vi "Keyence handler.vi"(8 "error in (no error)":errorcluster, 11 "Message Queues out":T3) -> (0 "error out":errorcluster, 3 "Message Queue":refnum<queue>)   [LabVIEW 2014]
uses:
  support/Message Queue/All Message Queues.ctl
  support/Message Queue/Message Cluster.ctl
  Keyence data cluster.ctl
  Keyence Status.ctl
  support/Message Queue/Lossy Enqueue Message (Single).vi
  support/Message Queue/Enqueue Message (Single).vi
  <vilib>/Utility/error.llb/Error Cluster From Error Code.vi
  <vilib>/ErrorRing/Error Ring.xnode
  support/Message Queue/Message Queue.lvlib
panel:
  in  "MBActX":refnum<k7>(container)
  out "Keyence Data Cluster":T1
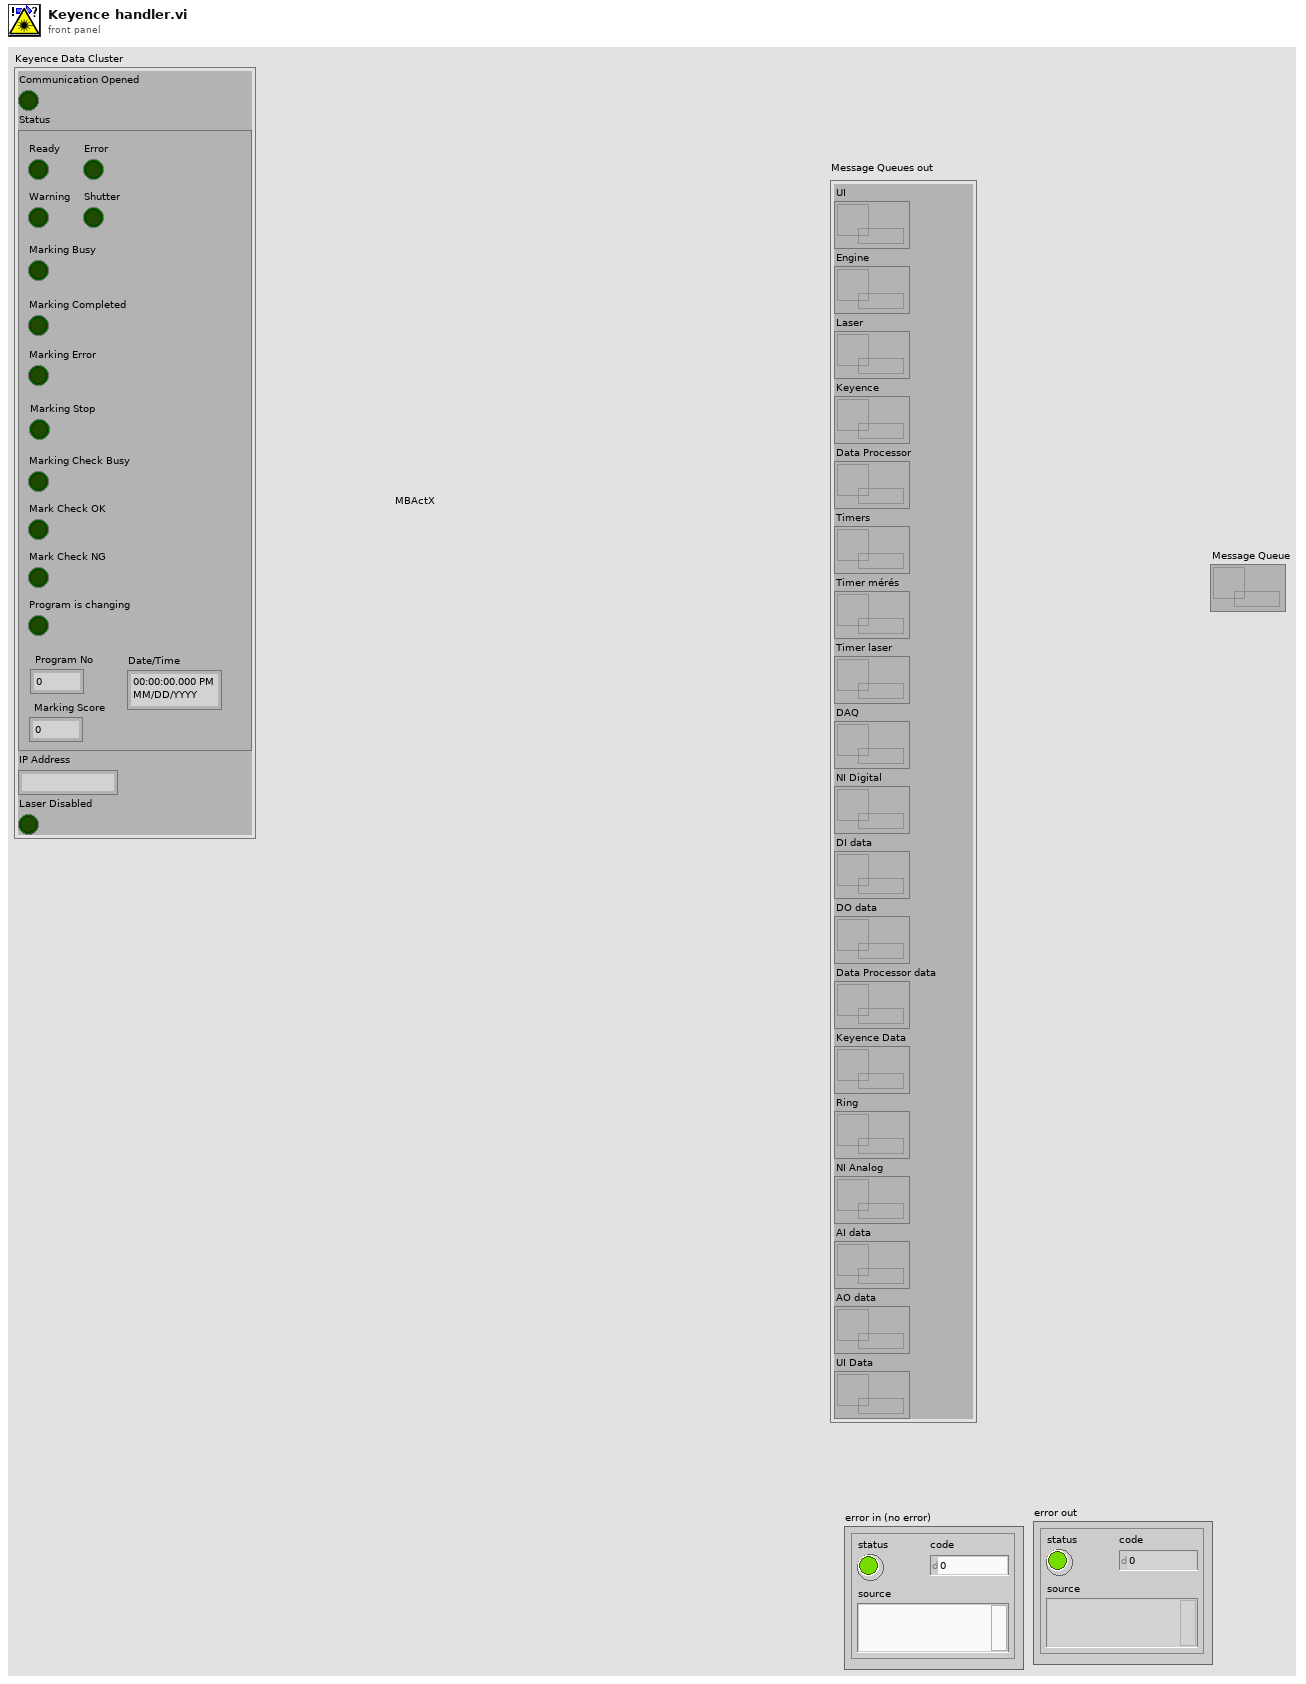
[diagram p1: front panel]
types:
  T1 = typedef "Keyence data cluster.ctl" = cluster{"Communication Opened":bool, "Status":T2, "IP Address":string, "Laser Disabled":bool}
  T2 = typedef "Keyence Status.ctl" = cluster{"Ready":bool, "Error":bool, "Warning":bool, "Shutter":bool, "Mark Check OK":bool, "Mark Check NG":bool, "Marking Busy":bool, "Program No":u16, "Marking Check Busy":bool, "Marking Completed":bool, "Marking Score":u16, "Marking Error":bool, "Marking Stop":bool, "Program is changing":bool, "Date/Time":timestamp}
  T3 = typedef "Message Queue.lvlib/All Message Queues.ctl" = cluster{"UI":refnum<queue>, "Engine":refnum<queue>, "Laser":refnum<queue>, "Keyence":refnum<queue>, "Data Processor":refnum<queue>, "Timers":refnum<queue>, "Timer mérés":refnum<queue>, "Timer laser":refnum<queue>, "DAQ":refnum<queue>, "NI Digital":refnum<queue>, "DI data":refnum<queue>, "DO data":refnum<queue>, "Data Processor data":refnum<queue>, "Keyence Data":refnum<queue>, "Ring":refnum<queue>, "NI Analog":refnum<queue>, "AI data":refnum<queue>, "AO data":refnum<queue>, "UI Data":refnum<queue>}
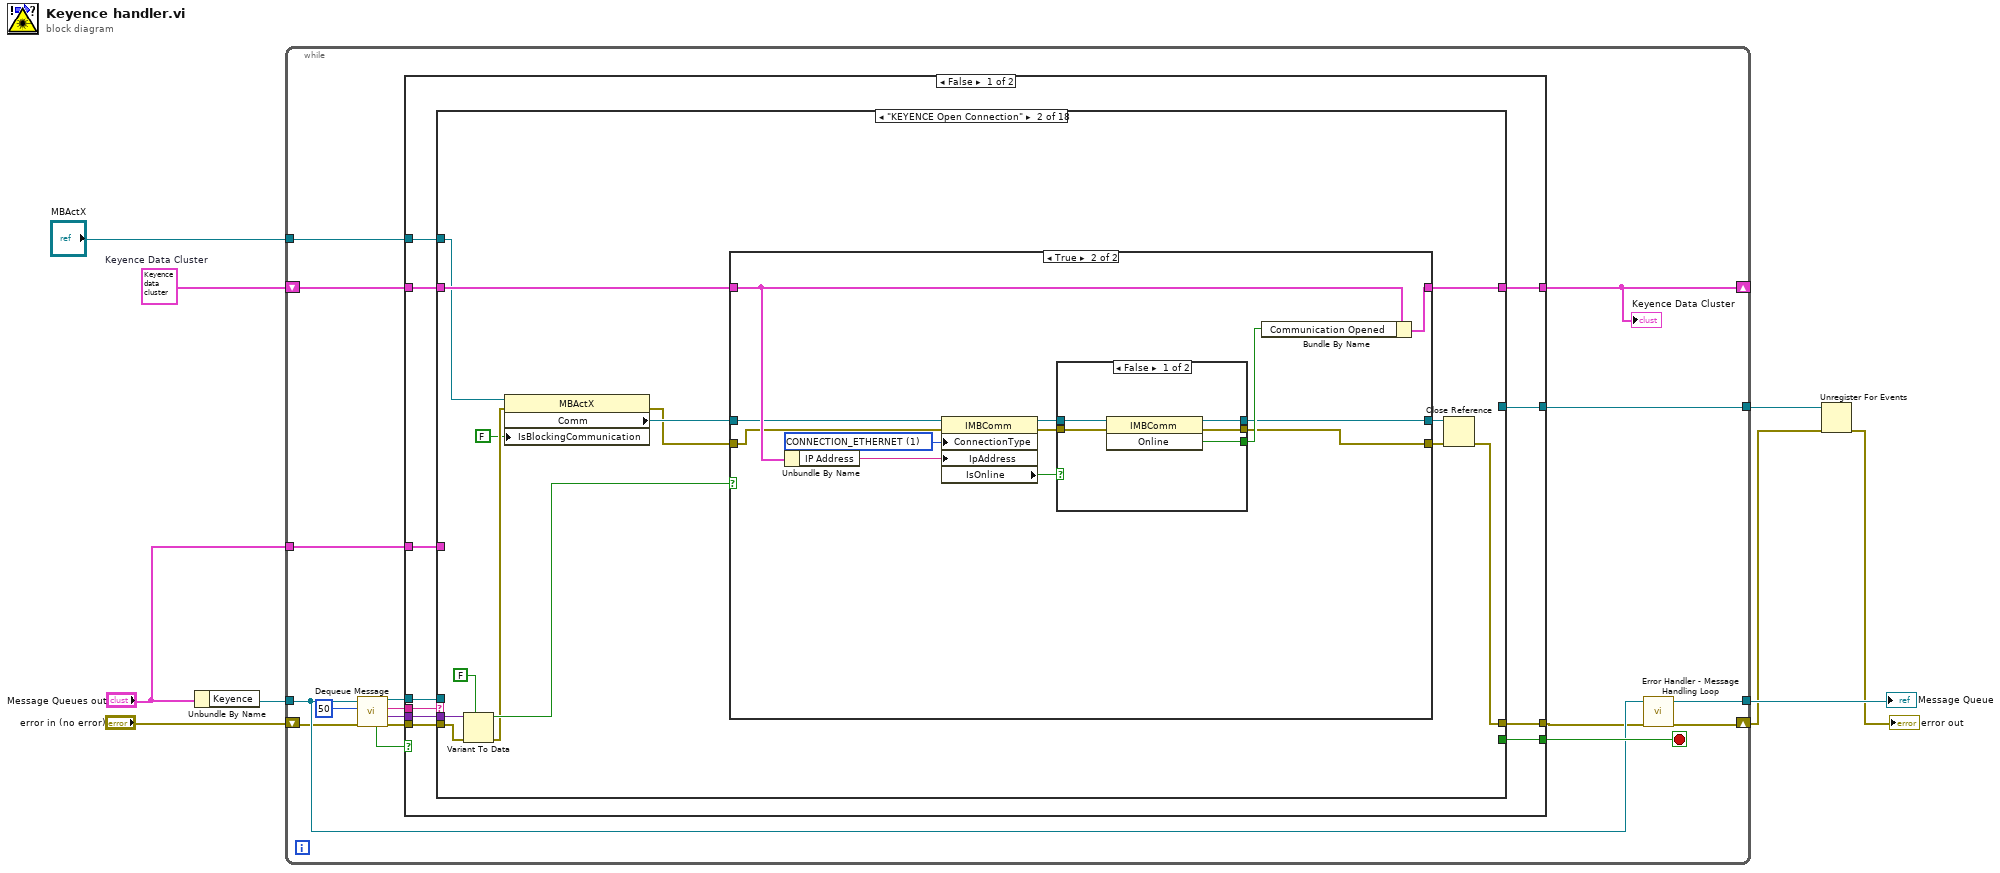
[diagram p0: block diagram]
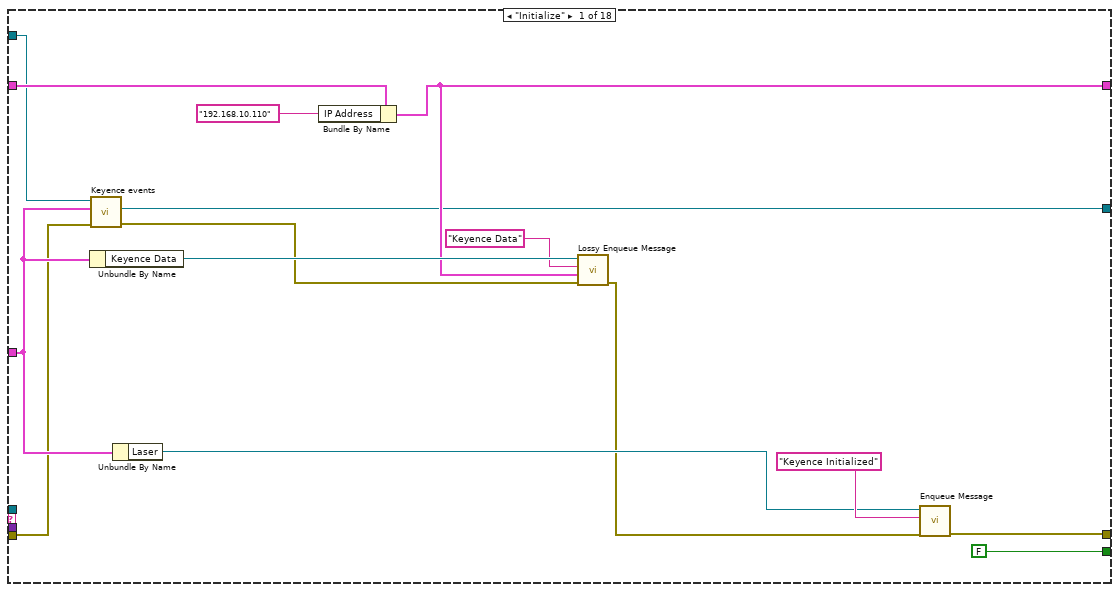
[diagram p2: hidden frame]
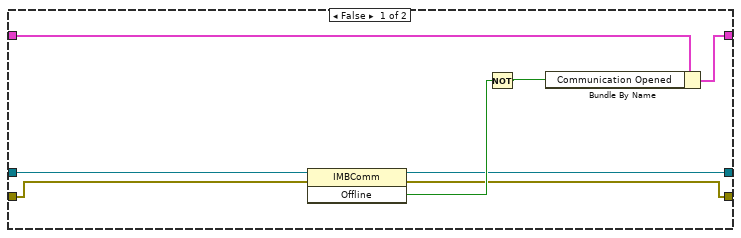
[diagram p3: hidden frame]
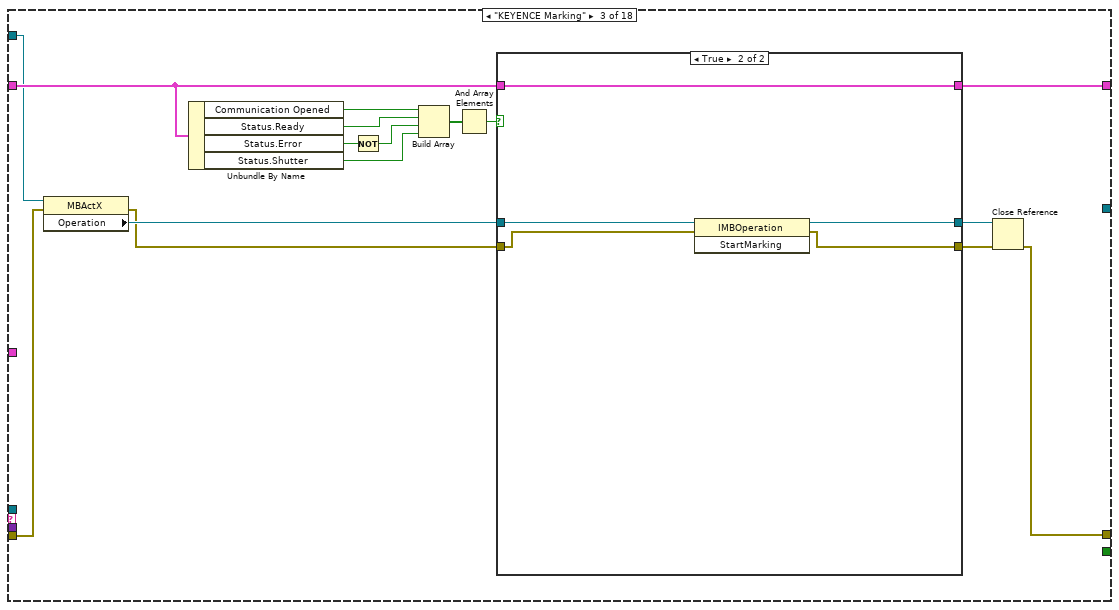
[diagram p5: hidden frame]
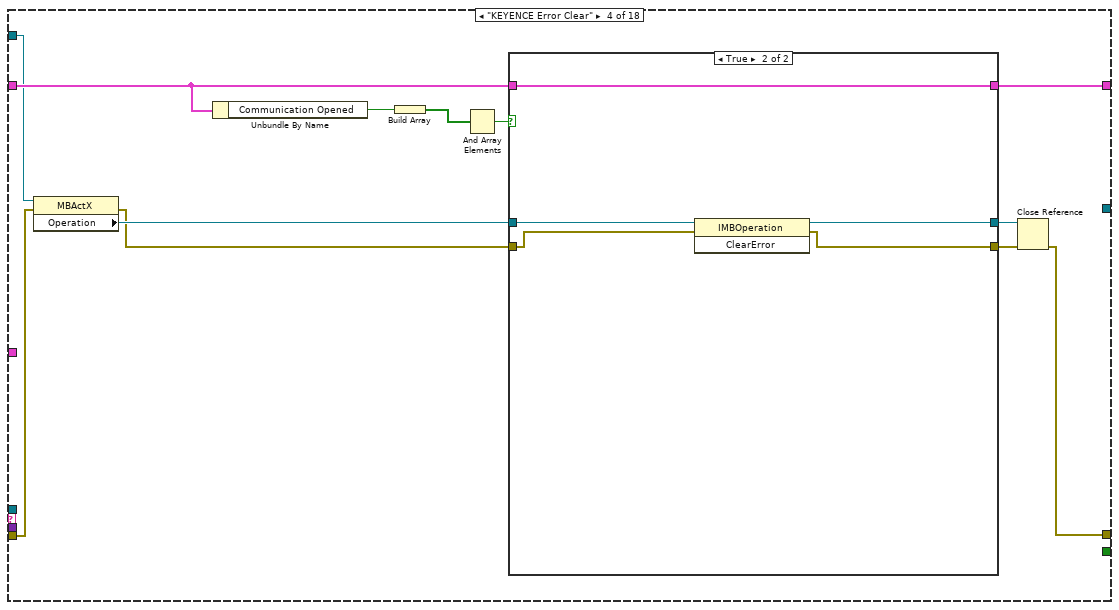
[diagram p7: hidden frame]
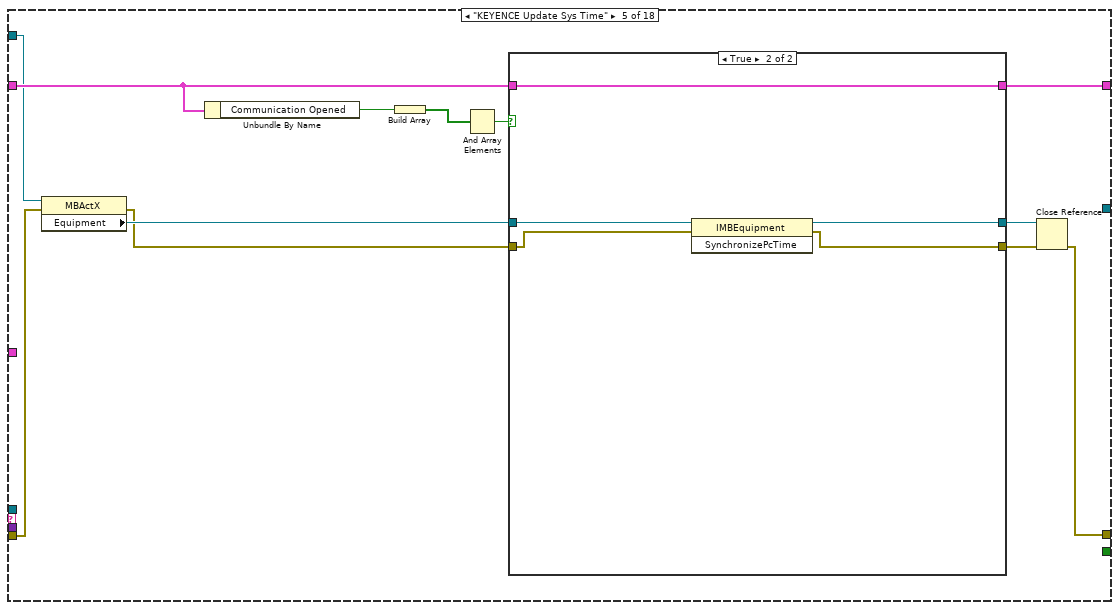
[diagram p9: hidden frame]
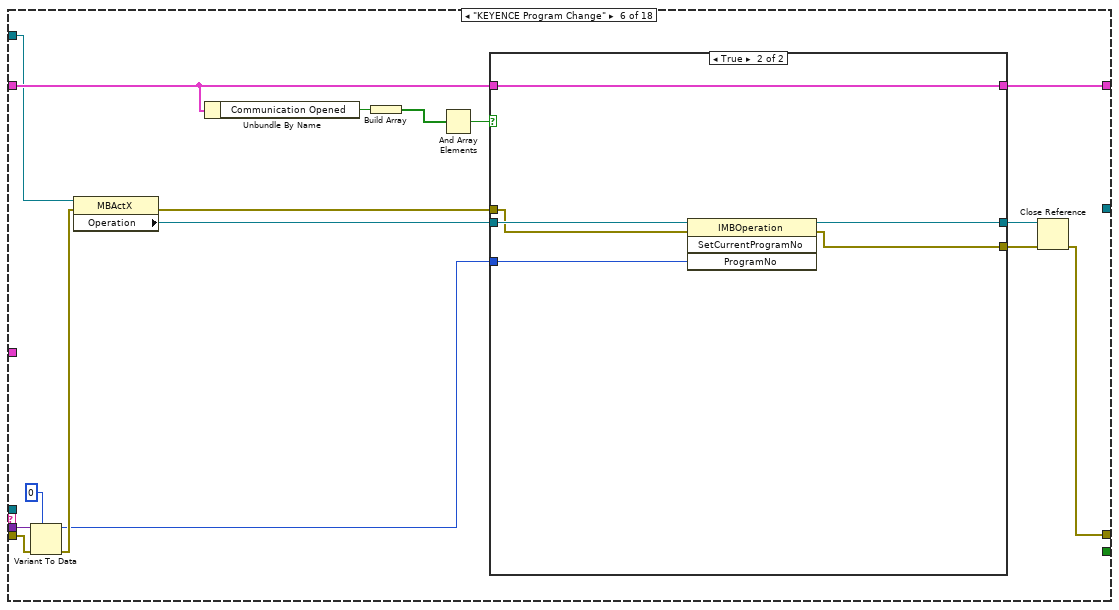
[diagram p11: hidden frame]
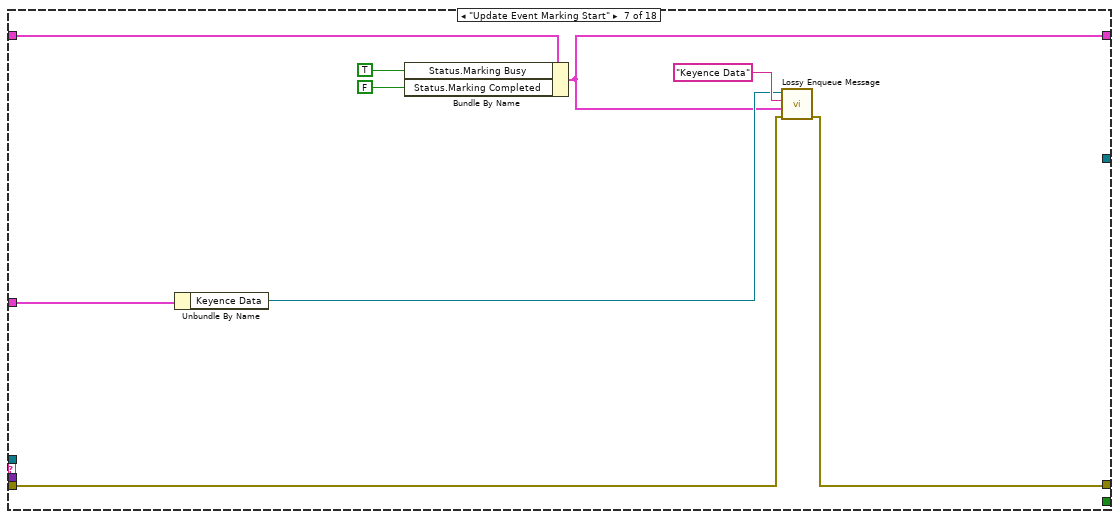
[diagram p13: hidden frame]
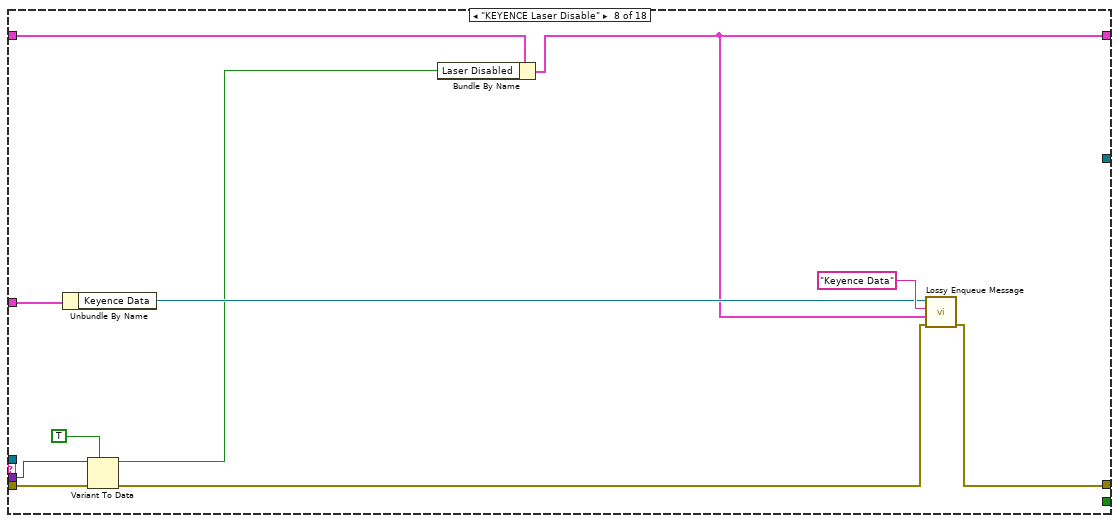
[diagram p14: hidden frame]
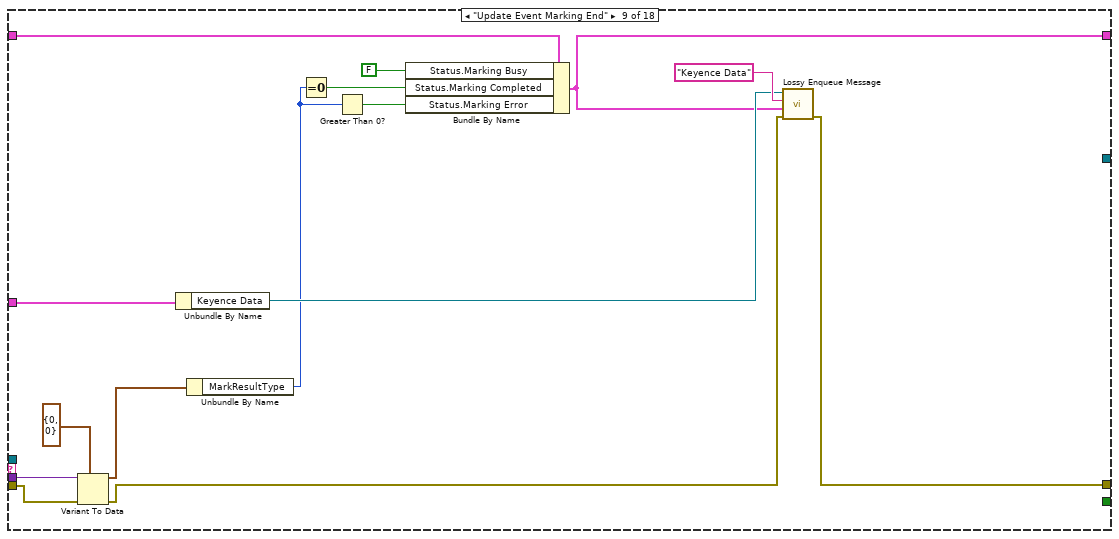
[diagram p15: hidden frame]
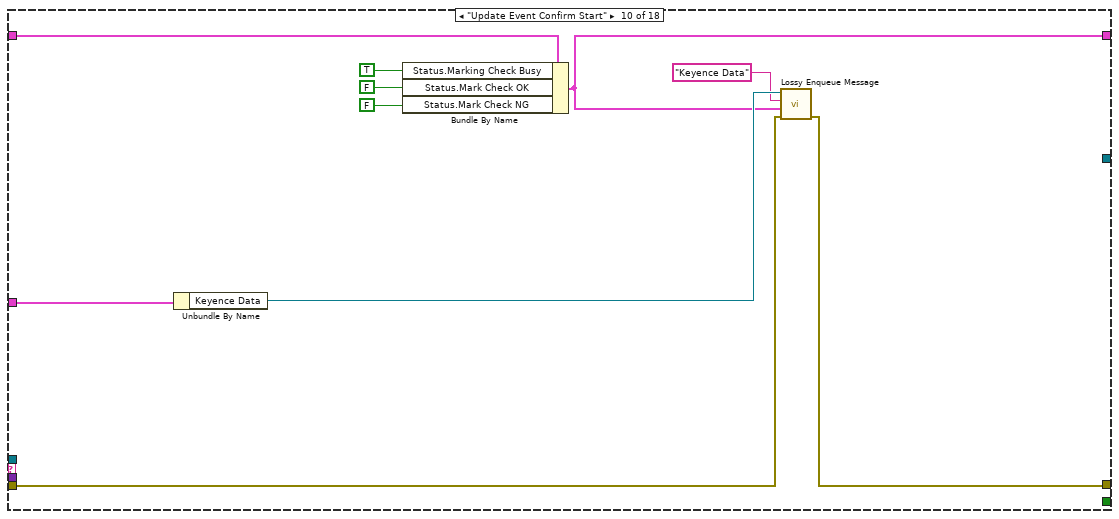
[diagram p16: hidden frame]
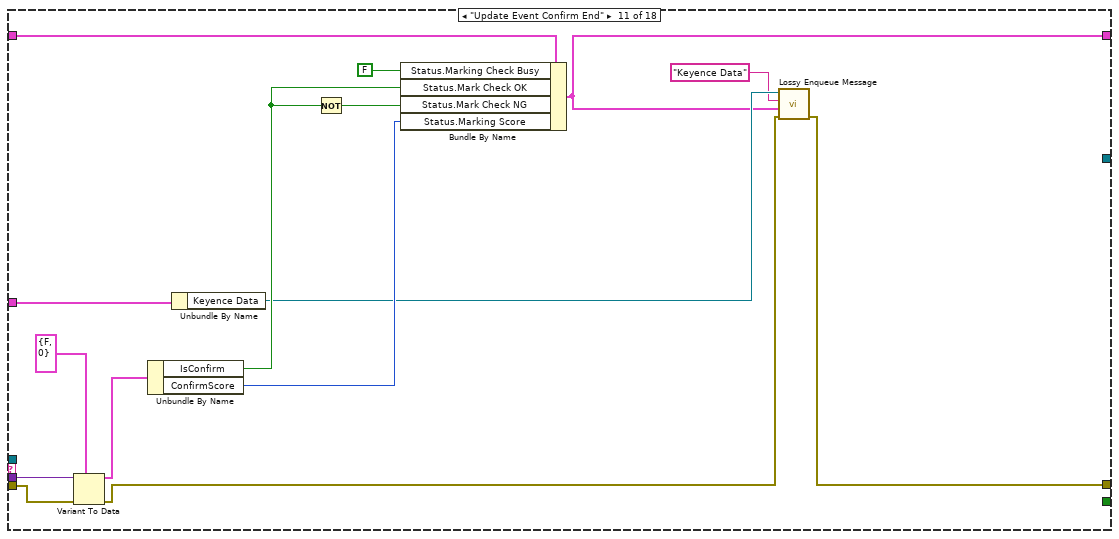
[diagram p17: hidden frame]
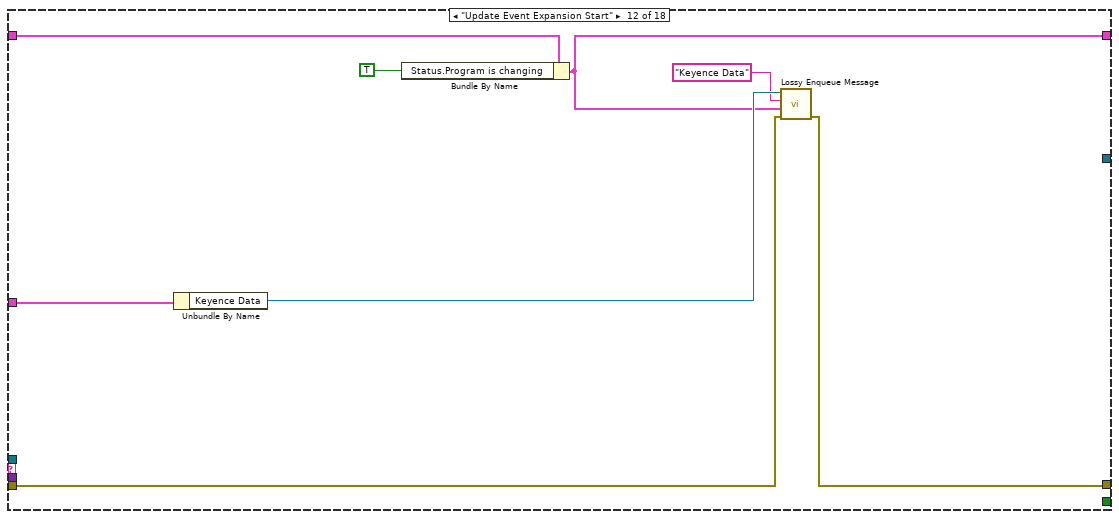
[diagram p18: hidden frame]
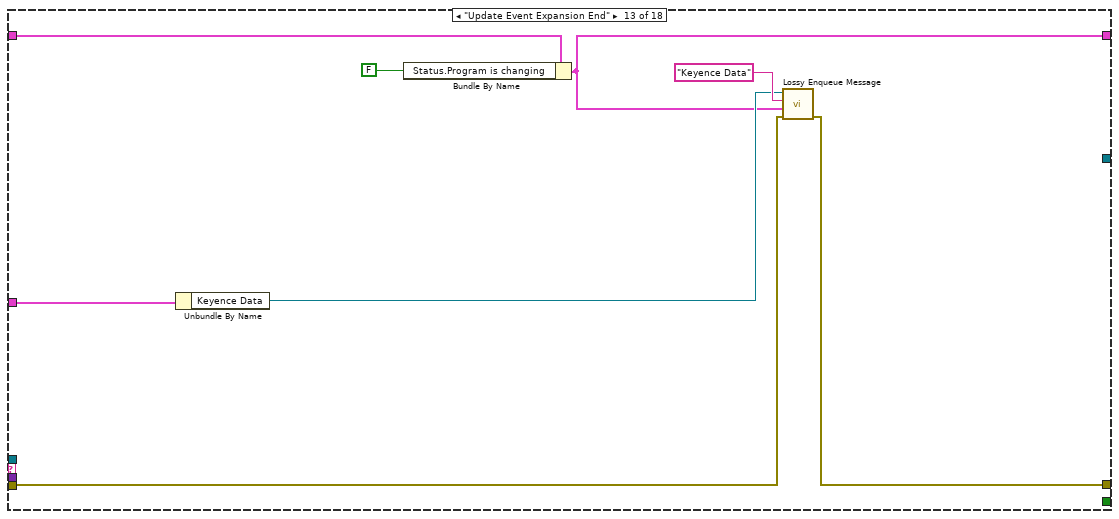
[diagram p19: hidden frame]
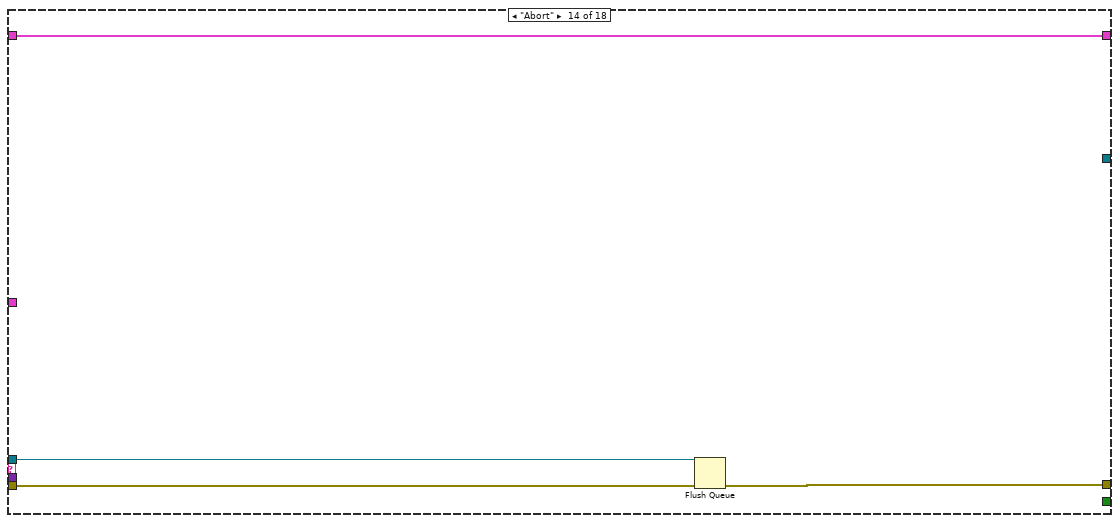
[diagram p20: hidden frame]
diagram:
  w6 = T1 {"Communication Opened"=FALSE, "Status"={"Ready"=FALSE, "Error"=FALSE, "Warning"=FALSE, "Shutter"=FALSE, "Mark Check OK"=FALSE, "Mark Check NG"=FALSE, "Marking Busy"=FALSE, "Program No"=0, "Marking Check Busy"=FALSE, "Marking Completed"=FALSE, "Marking Score"=0, "Marking Error"=FALSE, "Marking Stop"=FALSE, "Program is changing"=FALSE, "Date/Time"=timestamp(0 s since 1904-01-01)}, "IP Address"="", "Laser Disabled"=FALSE}  # Keyence Data Cluster
  n1 = Unbundle By Name("Message Queues out") -> ("Keyence"=w8:refnum<queue>)
  n2 = while {
    tunnel: w8 -> [w16]
    shift-right: [w15] -> _
    shift-left: w6 -> [w14]
    shift-right: [w19] -> w1
    shift-left: "error in (no error)" -> [w12]
    tunnel: "Message Queues out" -> [w18]
    tunnel: [w17] -> w7
    tunnel: [w13] -> w4
    tunnel: "MBActX" -> [w10]
    stop <- w23 stop-if-true
    n3 = call "Dequeue Message.vi"("error in (no error)"=w12, "timeout in ms (-1)"=50, "Message Queue"=w16) -> ("error out"=w25:errorcluster, "Message Data"=w20:variant, "Message"=w26:string, "dup Message Queue"=w24:refnum<queue>, "timed out?"=w21:bool)  [unwired: 4 in]
    n4 = case shown="False" w21 {
      tunnel: w26 -> [w37 _]
      tunnel: w25 -> [w36 w311]
      tunnel: w24 -> [w35 _]
      tunnel: [w34 FALSE] -> w23
      tunnel: [w33 w312] -> w11
      tunnel: w14 -> [w32 w310]
      tunnel: [w29 w306] -> w15
      tunnel: w20 -> [w31 _]
      tunnel: w18 -> [w30 w308]
      tunnel: w10 -> [w28 w304]
      tunnel: [w27 _] -> w13
      frame False {
        n5 = case shown="\"KEYENCE Open Connection\"" w37 {
          selector: w37 -> [_ _ _ _ _ _ _ _ _ _ _ _ _ _ _ _ _ w293]
          tunnel: w36 -> [w41 w63 w101 w125 w145 w167 w185 w196 w206 w220 w231 w245 w253 w263 w265 w279 w282 _]
          tunnel: w35 -> [_ _ _ _ _ _ _ _ _ _ _ _ _ w262 w268 w278 w292 _]
          tunnel: [w51 w54 w98 w121 w141 w161 w184 w198 w204 w219 w229 w244 w252 w260 w269 w280 w283 w294] -> w33
          tunnel: [FALSE _ _ _ _ _ _ _ _ _ _ _ _ _ _ _ TRUE FALSE] -> w34
          tunnel: w32 -> [w48 w62 w109 w129 w149 w173 w188 w201 w210 w223 w235 w248 w256 w261 w264 w281 w290 w296]
          tunnel: w31 -> [_ w64 _ _ _ w168 _ w195 w207 _ w232 _ _ _ w266 _ _ _]
          tunnel: w30 -> [w42 _ _ _ _ _ w186 w199 w208 w221 w233 w246 w254 _ w267 _ w285 _]
          tunnel: [w44 w61 w110 w130 w150 w174 w187 w200 w209 w222 w234 w247 w255 w261 w264 w281 w290 w296] -> w29
          tunnel: w28 -> [w38 w57 w100 w124 w144 w164 _ _ _ _ _ _ _ _ _ _ _ _]
          tunnel: [w39 _ _ _ _ _ _ _ _ _ _ _ _ _ _ _ _ _] -> w27
          frame "Initialize" {
            n6 = Unbundle By Name(w42) -> ("Keyence Data"=w46:refnum<queue>)
            n7 = call "Keyence events.vi"("error in"=w41, "Variant"=w42, "Automation Refnum in"=w38) -> ("error out"=w40:errorcluster, "event callback refnum"=w39:refnum<k27>)  [unwired: 7 in]
            n8 = Unbundle By Name(w42) -> ("Laser"=w49:refnum<queue>)
            n9 = Bundle By Name(cluster=w48, "IP Address"="192.168.10.110" ("Ethernet/IP parameters.Network path")) -> (w44:T1)
            n10 = call-poly "Lossy Enqueue Message.vi"("error in (no error)"=w40, "Message Data"=w44, "Message"="Keyence Data", "Message Queue"=w46) -> ("error out"=w43:errorcluster)  [unwired: 6 in, 1 out]
            n11 = call-poly "Enqueue Message.vi"("error in (no error)"=w43, "Message"="Keyence Initialized", "Message Queue"=w49) -> ("error out"=w51:errorcluster)  [unwired: 7 in, 1 out]
          }
          frame "KEYENCE Open Connection" {
            n12 = Variant To Data(error in=w63, type=FALSE ("Control word.Enable Voltage"), Variant=w64) -> (data=w65:bool, error out=w60:errorcluster)
            n13 = property class="MBActX"(reference=w57, error in=w60, "IsBlockingCommunication"=FALSE) -> (error out=w53:errorcluster, "Comm"=w58:refnum<k7>)  [unwired: 1 out]
            n14 = case shown="True" w65 {
              tunnel: w62 -> [w74 w86]
              tunnel: [w73 w85] -> w61
              tunnel: w58 -> [w72 w78]
              tunnel: w53 -> [w71 w77]
              tunnel: [w68 w76] -> w56
              tunnel: [w67 w75] -> w55
              frame False {
                n15 = invoke class="IMBComm" method="Offline"(reference=w72, error in=w71) -> (reference out=w68:refnum<k7>, error out=w67:errorcluster, "Offline"=w69:bool)  [unwired: 1 in]
                n16 = Not(x=w69) -> (.not. x?=w70:bool)
                n17 = Bundle By Name(cluster=w74, "Communication Opened"=w70) -> (w73:T1)
              }
              frame True {
                w84 = 1 items=["CONNECTION_USB", "CONNECTION_ETHERNET"] ("ConnectionType")
                n18 = Unbundle By Name(w86) -> ("IP Address"=w83:string)
                n19 = property class="IMBComm"(reference=w78, error in=w77, "ConnectionType"=w84, "IpAddress"=w83) -> (reference out=w82:refnum<k7>, error out=w79:errorcluster, "IsOnline"=w81:bool)
                n20 = case shown="False" w81 {
                  selector: w81 -> [_ w94]
                  tunnel: w82 -> [w91 w92]
                  tunnel: [w90 w94] -> w80
                  tunnel: w79 -> [w89 w93]
                  tunnel: [w88 w93] -> w75
                  tunnel: [w87 w92] -> w76
                  frame False {
                    n21 = invoke class="IMBComm" method="Online"(reference=w91, error in=w89) -> (reference out=w87:refnum<k7>, error out=w88:errorcluster, "Online"=w90:bool)  [unwired: 1 in]
                  }
                  frame True {
                  }
                }
                n22 = Bundle By Name(cluster=w86, "Communication Opened"=w80) -> (w85:T1)
              }
            }
            n23 = Close Reference(reference=w56, error in (no error)=w55) -> (error out=w54:errorcluster)
          }
          frame "KEYENCE Marking" {
            n24 = property class="MBActX"(reference=w100, error in=w101) -> (error out=w95:errorcluster, "Operation"=w96:refnum<k7>)  [unwired: 1 out]
            n25 = Unbundle By Name(w109) -> ("Communication Opened"=w107:bool, "Status.Ready"=w106:bool, "Status.Error"=w105:bool, "Status.Shutter"=w102:bool)
            n26 = Not(x=w105) -> (.not. x?=w103:bool)
            n27 = Build Array(w107, w106, w103, w102) -> (w104:bool[])
            n28 = And Array Elements(Boolean array=w104) -> (logical AND=w108:bool)
            n29 = case shown="True" w108 {
              tunnel: w109 -> [w113 w118]
              tunnel: [w113 w118] -> w110
              tunnel: w96 -> [w111 w117]
              tunnel: w95 -> [w112 w116]
              tunnel: [w111 w115] -> w99
              tunnel: [w112 w114] -> w97
              frame False {
              }
              frame True {
                n30 = invoke class="IMBOperation" method="StartMarking"(reference=w117, error in=w116) -> (reference out=w115:refnum<k7>, error out=w114:errorcluster)  [unwired: 1 in, 1 out]
              }
            }
            n31 = Close Reference(reference=w99, error in (no error)=w97) -> (error out=w98:errorcluster)
          }
          frame "KEYENCE Error Clear" {
            n32 = property class="MBActX"(reference=w124, error in=w125) -> (error out=w119:errorcluster, "Operation"=w120:refnum<k7>)  [unwired: 1 out]
            n33 = Unbundle By Name(w129) -> ("Communication Opened"=w127:bool)
            n34 = Build Array(w127) -> (w126:bool[])
            n35 = And Array Elements(Boolean array=w126) -> (logical AND=w128:bool)
            n36 = case shown="True" w128 {
              tunnel: w129 -> [w133 w138]
              tunnel: [w133 w138] -> w130
              tunnel: w120 -> [w131 w137]
              tunnel: w119 -> [w132 w136]
              tunnel: [w131 w135] -> w123
              tunnel: [w132 w134] -> w122
              frame False {
              }
              frame True {
                n37 = invoke class="IMBOperation" method="ClearError"(reference=w137, error in=w136) -> (reference out=w135:refnum<k7>, error out=w134:errorcluster)  [unwired: 1 in, 1 out]
              }
            }
            n38 = Close Reference(reference=w123, error in (no error)=w122) -> (error out=w121:errorcluster)
          }
          frame "KEYENCE Update Sys Time" {
            n39 = property class="MBActX"(reference=w144, error in=w145) -> (error out=w139:errorcluster, "Equipment"=w140:refnum<k7>)  [unwired: 1 out]
            n40 = Unbundle By Name(w149) -> ("Communication Opened"=w147:bool)
            n41 = Build Array(w147) -> (w146:bool[])
            n42 = And Array Elements(Boolean array=w146) -> (logical AND=w148:bool)
            n43 = case shown="True" w148 {
              tunnel: w149 -> [w153 w158]
              tunnel: [w153 w158] -> w150
              tunnel: w140 -> [w152 w157]
              tunnel: w139 -> [w151 w156]
              tunnel: [w152 w155] -> w143
              tunnel: [w151 w154] -> w142
              frame False {
              }
              frame True {
                n44 = invoke class="IMBEquipment" method="SynchronizePcTime"(reference=w157, error in=w156) -> (reference out=w155:refnum<k7>, error out=w154:errorcluster)  [unwired: 1 in, 1 out]
              }
            }
            n45 = Close Reference(reference=w143, error in (no error)=w142) -> (error out=w141:errorcluster)
          }
          frame "KEYENCE Program Change" {
            n46 = Variant To Data(error in=w167, type=u16 0, Variant=w168) -> (data=w165:u16, error out=w166:errorcluster)
            n47 = property class="MBActX"(reference=w164, error in=w166) -> (error out=w159:errorcluster, "Operation"=w160:refnum<k7>)  [unwired: 1 out]
            n48 = Unbundle By Name(w173) -> ("Communication Opened"=w171:bool)
            n49 = Build Array(w171) -> (w170:bool[])
            n50 = And Array Elements(Boolean array=w170) -> (logical AND=w172:bool)
            n51 = case shown="True" w172 {
              tunnel: w173 -> [w177 w183]
              tunnel: [w177 w183] -> w174
              tunnel: w160 -> [w176 w182]
              tunnel: w159 -> [w175 w181]
              tunnel: w165 -> [_ w180]
              tunnel: [w176 w179] -> w163
              tunnel: [w175 w178] -> w162
              frame False {
              }
              frame True {
                n52 = invoke class="IMBOperation" method="SetCurrentProgramNo"(reference=w182, error in=w181, "ProgramNo"=w180) -> (reference out=w179:refnum<k7>, error out=w178:errorcluster)  [unwired: 1 in, 2 out]
              }
            }
            n53 = Close Reference(reference=w163, error in (no error)=w162) -> (error out=w161:errorcluster)
          }
          frame "Update Event Marking Start" {
            n54 = Unbundle By Name(w186) -> ("Keyence Data"=w191:refnum<queue>)
            n55 = Bundle By Name(cluster=w188, "Status.Marking Busy"=TRUE, "Status.Marking Completed"=FALSE ("Status.Marking Busy")) -> (w187:T1)
            n56 = call-poly "Lossy Enqueue Message.vi"("error in (no error)"=w185, "Message Data"=w187, "Message"="Keyence Data", "Message Queue"=w191) -> ("error out"=w184:errorcluster)  [unwired: 6 in, 1 out]
          }
          frame "KEYENCE Laser Disable" {
            n57 = Unbundle By Name(w199) -> ("Keyence Data"=w202:refnum<queue>)
            n58 = Variant To Data(error in=w196, type=TRUE, Variant=w195) -> (data=w193:bool, error out=w194:errorcluster)
            n59 = Bundle By Name(cluster=w201, "Laser Disabled"=w193) -> (w200:T1)
            n60 = call-poly "Lossy Enqueue Message.vi"("error in (no error)"=w194, "Message Data"=w200, "Message"="Keyence Data", "Message Queue"=w202) -> ("error out"=w198:errorcluster)  [unwired: 6 in, 1 out]
          }
          frame "Update Event Marking End" {
            n61 = Variant To Data(error in=w206, type=cluster{"MarkResultType":i32, "MarkTime":i32} {"MarkResultType"=0, "MarkTime"=0} ("Event Data"), Variant=w207) -> (data=w214:cluster{"MarkResultType":i32, "MarkTime":i32}, error out=w205:errorcluster)
            n62 = Unbundle By Name(w208) -> ("Keyence Data"=w217:refnum<queue>)
            n63 = Unbundle By Name(w214) -> ("MarkResultType"=w211:i32)
            n64 = Equal To 0?(x=w211) -> (x = 0?=w213:bool)
            n65 = Greater Than 0?(x=w211) -> (x > 0?=w212:bool)
            n66 = Bundle By Name(cluster=w210, "Status.Marking Busy"=FALSE, "Status.Marking Completed"=w213, "Status.Marking Error"=w212) -> (w209:T1)
            n67 = call-poly "Lossy Enqueue Message.vi"("error in (no error)"=w205, "Message Data"=w209, "Message"="Keyence Data", "Message Queue"=w217) -> ("error out"=w204:errorcluster)  [unwired: 6 in, 1 out]
          }
          frame "Update Event Confirm Start" {
            n68 = Unbundle By Name(w221) -> ("Keyence Data"=w225:refnum<queue>)
            n69 = Bundle By Name(cluster=w223, "Status.Marking Check Busy"=TRUE ("Status.Marking Busy"), "Status.Mark Check OK"=FALSE ("Status.Marking Busy"), "Status.Mark Check NG"=FALSE ("Status.Marking Busy")) -> (w222:T1)
            n70 = call-poly "Lossy Enqueue Message.vi"("error in (no error)"=w220, "Message Data"=w222, "Message"="Keyence Data", "Message Queue"=w225) -> ("error out"=w219:errorcluster)  [unwired: 6 in, 1 out]
          }
          frame "Update Event Confirm End" {
            n71 = Variant To Data(error in=w231, type=cluster{"IsConfirm":bool, "ConfirmScore":i32} {"IsConfirm"=FALSE, "ConfirmScore"=0} ("Event Data"), Variant=w232) -> (data=w239:cluster{"IsConfirm":bool, "ConfirmScore":i32}, error out=w230:errorcluster)
            n72 = Unbundle By Name(w239) -> ("IsConfirm"=w243:bool, "ConfirmScore"=w241:i32)
            n73 = Unbundle By Name(w233) -> ("Keyence Data"=w237:refnum<queue>)
            n74 = Not(x=w243) -> (.not. x?=w242:bool)
            n75 = Bundle By Name(cluster=w235, "Status.Marking Check Busy"=FALSE ("Status.Marking Busy"), "Status.Mark Check OK"=w243, "Status.Mark Check NG"=w242, "Status.Marking Score"=w241) -> (w234:T1)
            n76 = call-poly "Lossy Enqueue Message.vi"("error in (no error)"=w230, "Message Data"=w234, "Message"="Keyence Data", "Message Queue"=w237) -> ("error out"=w229:errorcluster)  [unwired: 6 in, 1 out]
          }
          frame "Update Event Expansion Start" {
            n77 = Unbundle By Name(w246) -> ("Keyence Data"=w250:refnum<queue>)
            n78 = Bundle By Name(cluster=w248, "Status.Program is changing"=TRUE ("Status.Marking Busy")) -> (w247:T1)
            n79 = call-poly "Lossy Enqueue Message.vi"("error in (no error)"=w245, "Message Data"=w247, "Message"="Keyence Data", "Message Queue"=w250) -> ("error out"=w244:errorcluster)  [unwired: 6 in, 1 out]
          }
          frame "Update Event Expansion End" {
            n80 = Unbundle By Name(w254) -> ("Keyence Data"=w258:refnum<queue>)
            n81 = Bundle By Name(cluster=w256, "Status.Program is changing"=FALSE ("Status.Marking Busy")) -> (w255:T1)
            n82 = call-poly "Lossy Enqueue Message.vi"("error in (no error)"=w253, "Message Data"=w255, "Message"="Keyence Data", "Message Queue"=w258) -> ("error out"=w252:errorcluster)  [unwired: 6 in, 1 out]
          }
          frame "Abort" {
            n83 = Flush Queue(queue=w262, error in (no error)=w263) -> (error out=w260:errorcluster)  [unwired: 2 out]
          }
          frame "Error" {
            n84 = Unbundle By Name(w267) -> ("UI"=w272:refnum<queue>)
            n85 = call-poly "Enqueue Message.vi"("error in (no error)"=w265, "Message Data"=w266, "Message"="Error", "Message Queue"=w272) -> ("error out"=w274:errorcluster)  [unwired: 6 in, 1 out]
            n86 = call-poly "Enqueue Message.vi"("Priority Message? (F)"=TRUE, "error in (no error)"=w265, "Message"="Initiate Stop", "Message Queue"=w268) -> ("error out"=w273:errorcluster)  [unwired: 6 in, 1 out]
            n87 = Merge Errors(w274, w273) -> (w269:errorcluster)
          }
          frame "Initiate Stop" {
            n88 = call-poly "Enqueue Message.vi"("Priority Message? (F)"=TRUE, "error in (no error)"=w279, "Message"="Program Stop", "Message Queue"=w278) -> ("error out"=w280:errorcluster)  [unwired: 6 in, 1 out]
          }
          frame "Program Stop" {
            n89 = Flush Queue(queue=w292, error in (no error)=w282) -> (error out=w284:errorcluster)  [unwired: 2 out]
            n90 = Unbundle By Name(w285) -> ("Keyence Data"=w286:refnum<queue>)
            n91 = Flush Queue(queue=w286, error in (no error)=w282) -> (queue out=w287:refnum<queue>, error out=w288:errorcluster)  [unwired: 1 out]
            n92 = Release Queue(queue=w287, error in (no error)=w288) -> (error out=w289:errorcluster)  [unwired: 1 in, 2 out]
            n93 = Merge Errors(w289, w284) -> (w283:errorcluster)
          }
          frame Default {
            n94 = xnode "Error Ring"("parameter 0"=w293) -> ("error out"=w294:errorcluster)
          }
        }
      }
      frame True {
        n95 = Unbundle By Name(w310) -> ("Status"=w305:T2, "Communication Opened"=w309:bool)
        n96 = Unbundle By Name(w308) -> ("Keyence Data"=w307:refnum<queue>)
        n97 = case shown="True" w309 {
          tunnel: [w315 w327] -> w312
          tunnel: w311 -> [w316 w322]
          tunnel: w310 -> [w317 w326]
          tunnel: w307 -> [w314 w321]
          tunnel: [w317 w325] -> w306
          tunnel: w305 -> [_ w324]
          tunnel: w304 -> [_ w323]
          frame False {
            n98 = call-poly "Lossy Enqueue Message.vi"("error in (no error)"=w316, "Message Data"=w317, "Message"="Keyence Data", "Message Queue"=w314) -> ("error out"=w315:errorcluster)  [unwired: 6 in, 1 out]
          }
          frame True {
            n99 = call "Keyence ActiveX TimeOut.vi"("error in (no error)"=w322, "Status in"=w324, "Automation Refnum in"=w323) -> ("error out"=w319:errorcluster, "Status out"=w320:T2)  [unwired: 7 in]
            n100 = Bundle By Name(cluster=w326, "Status"=w320) -> (w325:T1)
            n101 = call-poly "Lossy Enqueue Message.vi"("error in (no error)"=w319, "Message Data"=w325, "Message"="Keyence Data", "Message Queue"=w321) -> ("error out"=w327:errorcluster)  [unwired: 6 in, 1 out]
          }
        }
      }
    }
    "Keyence Data Cluster" <- w15
    n102 = call "Error Handler - Message Handling Loop.vi"("error in (no error)"=w11, "Message Queue"=w16) -> ("dup error in"=w19:errorcluster, "dup Message Queue"=w17:refnum<queue>)  [unwired: 8 in]
  }
  "Message Queue" <- w7
  n103 = Unregister For Events(event registration refnum=w4, error in=w1) -> (error out=→"error out":errorcluster)
